vi "Get BLISS_Random Reject Image List (SubVI).vi"(5 "Reject Codes":string[](array[string])=["325", "326", "066", "067"], 7 "Save to Folder":path, 8 "error in":errorcluster, 9 "views search criteria":string, 10 "BLISS Server name":string, 11 "Number of Images Requested":i32=1) -> (0 "error out":errorcluster, 3 "Random File List":string[](array[string]))   [LabVIEW 2018]
panel:
  out "error out file save":errorcluster
  out "count":i32
  out "matched view":string
  out "filenames":string[](array[string])
  out "Reject Code":string
  out "View":string
  out "date":string
  out "Reject Codes for this View":string[](array[string])
  out "dates on this server":string[](array[string])
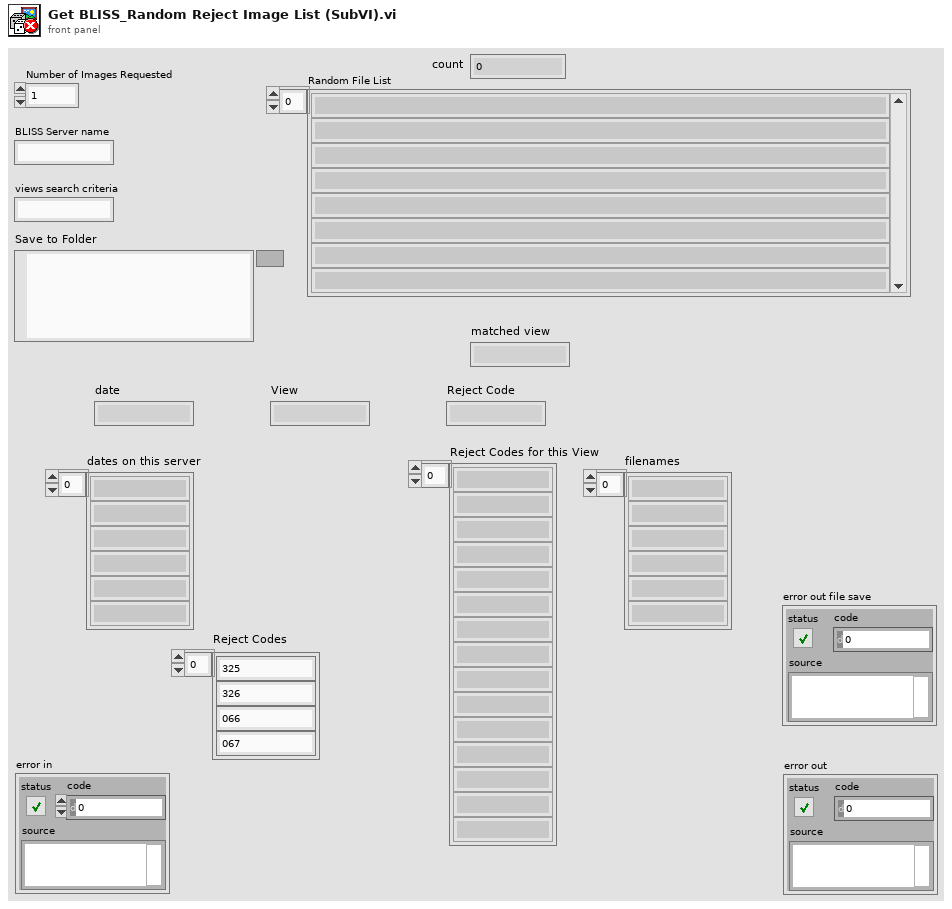
[diagram p1: front panel]
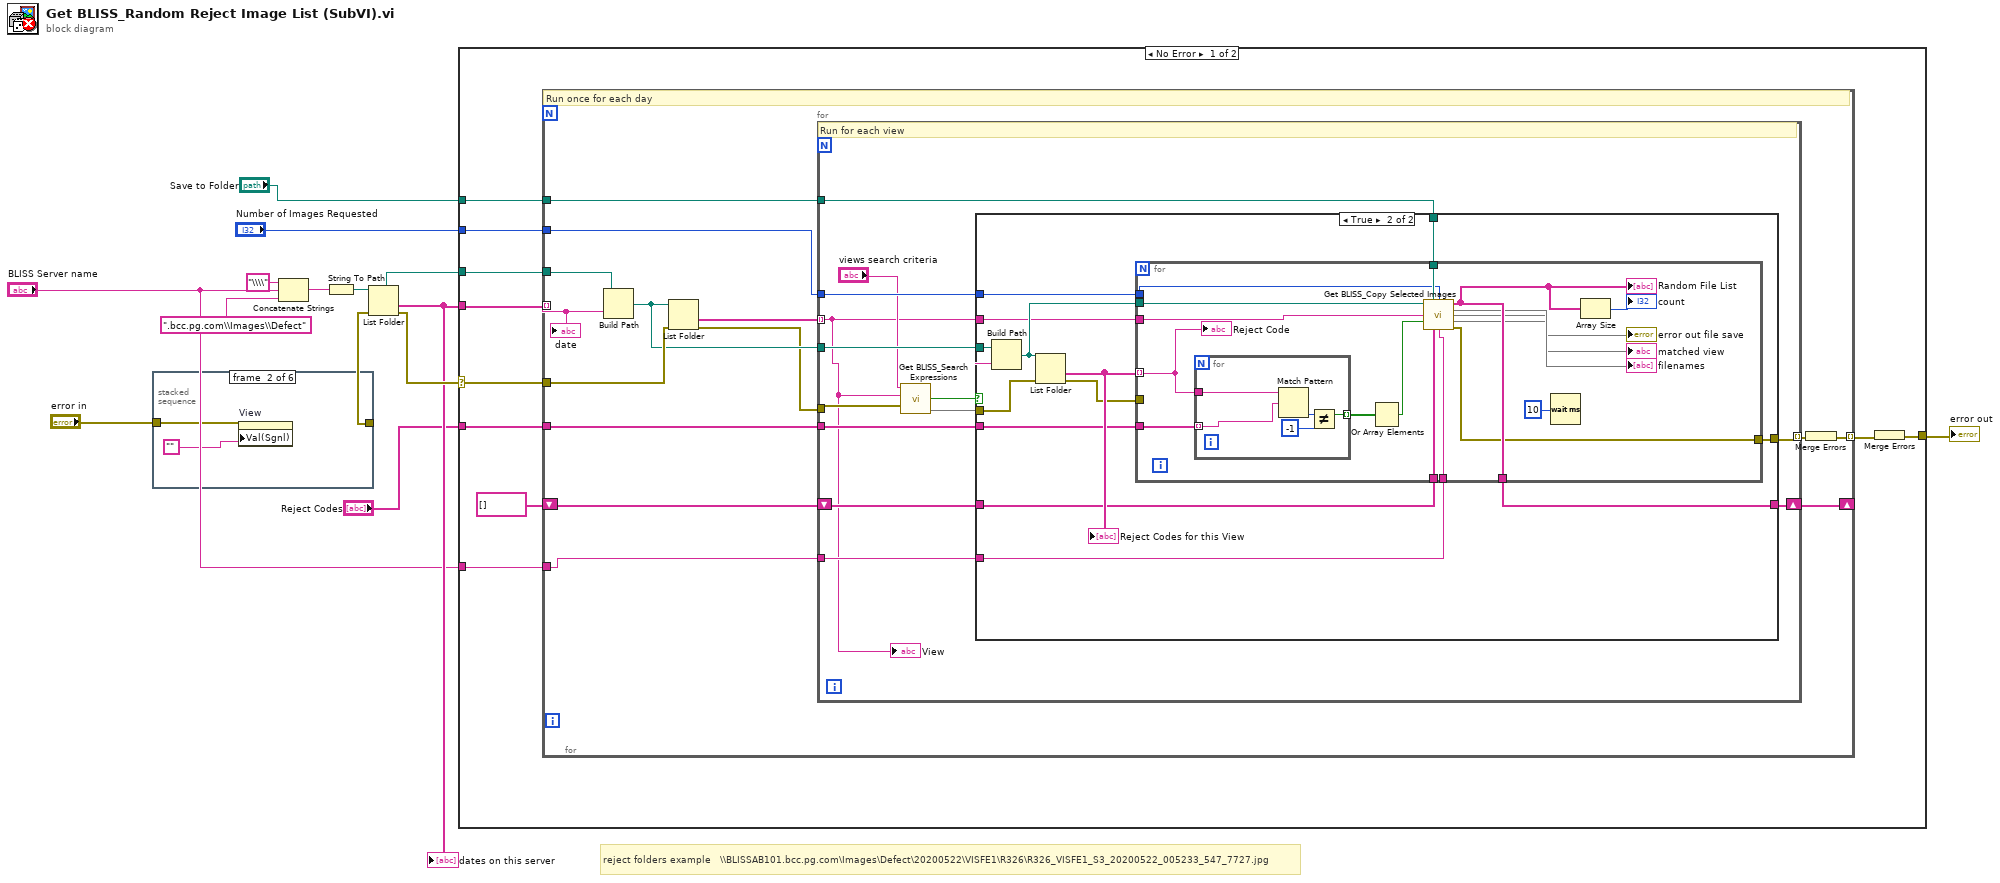
[diagram p0: block diagram]
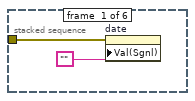
[diagram p2: hidden frame]
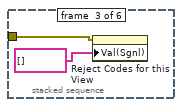
[diagram p3: hidden frame]
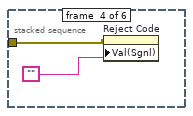
[diagram p4: hidden frame]
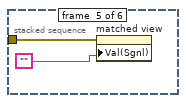
[diagram p5: hidden frame]
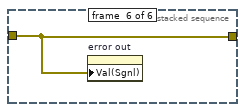
[diagram p6: hidden frame]
diagram:
  # "reject folders example   \\\\BLISSAB101.bcc.pg.com\\Images\\Defect\\20200522\\VISFE1\\R326\\R326_VISFE1_S3_20200522_005233_547_7727.jpg"
  n1 = stacked-sequence {
    tunnel: "error in" -> [w15 w16 w18 w20 w22 w24]
    tunnel: [_ _ _ _ _ w24] -> w4
    frame #0 {
      n2 = property on="date" class="Str"(error in=w15, "Val(Sgnl)"="") -> ()  [unwired: 1 in, 2 out]
    }
    frame #1 {
      n3 = property on="View" class="Str"(error in=w16, "Val(Sgnl)"="") -> ()  [unwired: 1 in, 2 out]
    }
    frame #2 {
      n4 = property on="Reject Codes for this View" class="Arr (strict)"(error in=w18, "Val(Sgnl)"=string[] [] ("Value (Signaling)")) -> ()  [unwired: 1 in, 2 out]
    }
    frame #3 {
      n5 = property on="Reject Code" class="Str"(error in=w20, "Val(Sgnl)"="") -> ()  [unwired: 1 in, 2 out]
    }
    frame #4 {
      n6 = property on="matched view" class="Str"(error in=w22, "Val(Sgnl)"="") -> ()  [unwired: 1 in, 2 out]
    }
    frame #5 {
      n7 = property on="error out" class="Clust (strict)"("Val(Sgnl)"=w24) -> ()  [unwired: 2 in, 2 out]
    }
  }
  n8 = Concatenate Strings("\\\\" ("string"), "BLISS Server name", ".bcc.pg.com\\Images\\Defect" ("string")) -> (w11:string)
  n9 = String To Path(string=w11) -> (path=w12:path)
  n10 = List Folder(path=w12, error in=w4) -> (folder names=w10:string[], error out=w13:errorcluster)  [unwired: 2 in, 2 out]
  "dates on this server" <- w10
  n11 = case shown="No Error" w13 {
    selector: w13 -> [w33 w98]
    tunnel: w10 -> [w32 _]
    tunnel: w12 -> [w34 _]
    tunnel: [w30 w98] -> w9
    tunnel: "BLISS Server name" -> [w28 _]
    tunnel: "Number of Images Requested" -> [w27 _]
    tunnel: "Save to Folder" -> [w26 _]
    tunnel: "Reject Codes" -> [w25 _]
    frame No Error {
      n12 = for {
        tunnel: w34 -> [w48]
        tunnel: w33 -> [w47]
        tunnel: [w46] -> w31 mode=indexing
        tunnel: w32 -> [w42] mode=indexing
        shift-right: [w41] -> _
        shift-left: string[] [] -> [w35]
        tunnel: w28 -> [w39]
        tunnel: w27 -> [w38]
        tunnel: w26 -> [w37]
        tunnel: w25 -> [w36]
        # "Run once for each day"
        n13 = Build Path(base path=w48, name or relative path=w42) -> (appended path=w45:path)
        n14 = List Folder(path=w45, error in=w47) -> (folder names=w40:string[], error out=w44:errorcluster)  [unwired: 2 in, 2 out]
        n15 = for {
          tunnel: w40 -> [w49] mode=indexing
          tunnel: w45 -> [w61]
          tunnel: w44 -> [w53]
          tunnel: [w57] -> w43 mode=indexing
          shift-right: [w58] -> w41
          shift-left: w35 -> [w54]
          tunnel: w38 -> [w60]
          tunnel: w39 -> [w59]
          tunnel: w37 -> [w56]
          tunnel: w36 -> [w55]
          # "Run for each view"
          n16 = call "Get BLISS_Search Expressions.vi"(8:w53, "String to Search"=w49, "Search Expressions\n(comma delimited)"="views search criteria") -> (0:w52, "Match?"=w51:bool)  [unwired: 6 in, 1 out]
          n17 = case shown="True" w51 {
            tunnel: w61 -> [_ w75]
            tunnel: w60 -> [_ w71]
            tunnel: w54 -> [w62 w70]
            tunnel: w59 -> [_ w69]
            tunnel: [w62 w68] -> w58
            tunnel: [_ w67] -> w57
            tunnel: w49 -> [_ w66]
            tunnel: w56 -> [_ w65]
            tunnel: w55 -> [_ w64]
            tunnel: w52 -> [_ w63]
            frame False {
            }
            frame True {
              n18 = Build Path(base path=w75, name or relative path=w66) -> (appended path=w72:path)
              n19 = List Folder(path=w72, error in=w63) -> (folder names=w74:string[], error out=w73:errorcluster)  [unwired: 2 in, 2 out]
              "Reject Codes for this View" <- w74
              n20 = for {
                tunnel: w74 -> [w78] mode=indexing
                tunnel: w72 -> [w91]
                tunnel: w65 -> [w90]
                tunnel: w71 -> [w89]
                tunnel: w66 -> [w76]
                tunnel: w70 -> [w88]
                tunnel: w69 -> [w87]
                tunnel: [w86] -> w68
                tunnel: [w84] -> w67
                tunnel: w73 -> [_]
                tunnel: w64 -> [w79]
                n21 = for {
                  tunnel: w78 -> [w97]
                  tunnel: w79 -> [w96] mode=indexing
                  tunnel: [w94] -> w80 mode=indexing
                  n22 = Match Pattern(string=w97, regular expression=w96) -> (offset past match=w95:i32)  [unwired: 1 in, 3 out]
                  n23 = Not Equal?(x=w95, y=-1) -> (x != y?=w94:bool)
                }
                n24 = Or Array Elements(Boolean array=w80) -> (logical OR=w77:bool)
                n25 = call "Get BLISS_Copy Selected Images.vi"("base path"=w91, 1:w90, 2:w89, 7:w76, "Valid"=w77, 12:w88, "BLISS Server name"=w87) -> ("Appended Image List"=w86:string[], 6:→"filenames", 8:→"matched view", 10:→"error out file save", "error out"=w84:errorcluster)  [unwired: 4 in]
                "Random File List" <- w86
                n26 = Wait (ms)(milliseconds to wait=u32 10) -> ()  [unwired: 1 out]
                n27 = Array Size(array=w86) -> (size(s)=→"count":i32)
                "Reject Code" <- w78
              }
            }
          }
          "View" <- w49
        }
        n28 = Merge Errors(w43) -> (w46:errorcluster)
        "date" <- w42
      }
      n29 = Merge Errors(w31) -> (w30:errorcluster)
    }
    frame Error {
    }
  }
  "error out" <- w9
